vi "ChirpData.vi"(6 "element":T1, 8 "error in (no error)":errorcluster, 9 "NumDataPoints":u32, 10 "Work Unit Data Points":csg[](array[numeric]), 11 "SETI_LV_FPGA in":refnum<class "SETI_LV_FPGA.lvclass">) -> (0 "error out":errorcluster, 1 "NumDataPoints":u32, 2 "ChirpedData out":csg[](array[numeric]), 3 "SETI_LV_FPGA out":refnum<class "SETI_LV_FPGA.lvclass">)   [LabVIEW 2015, in "SETI_LV_FPGA.lvclass"]
uses:
  SETI_LV_FPGA.lvclass
  SETI_LV/TypeDefs/ChirpFFT Pairs.ctl
  SETI_LV/SETI_LV.lvlib
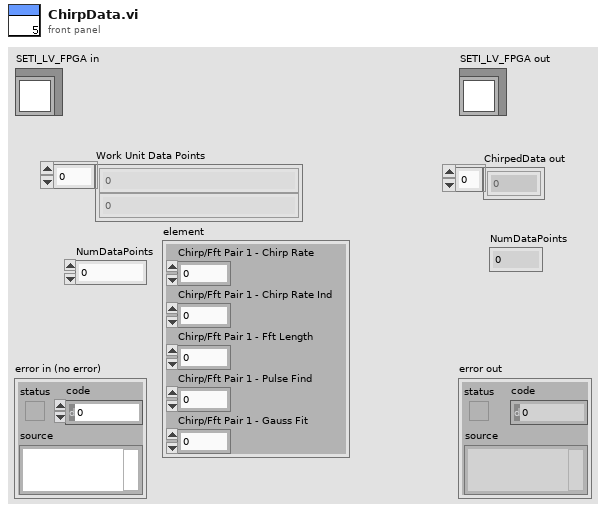
[diagram p1: front panel]
types:
  T1 = typedef "SETI_LV.lvlib/ChirpFFT Pairs.ctl" = cluster{"Chirp/Fft Pair 1 - Chirp Rate":dbl, "Chirp/Fft Pair 1 - Chirp Rate Ind":i32, "Chirp/Fft Pair 1 - Fft Length":i32, "Chirp/Fft Pair 1 - Pulse Find":i32, "Chirp/Fft Pair 1 - Gauss Fit":i32}
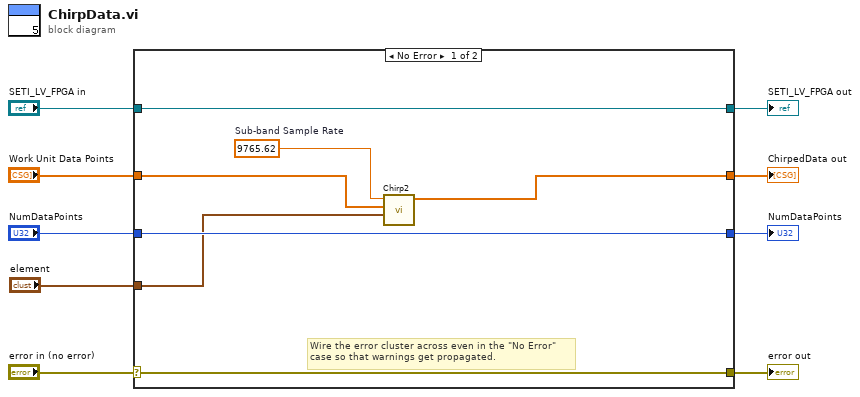
[diagram p0: block diagram]
diagram:
  n1 = case shown="No Error" "error in (no error)" {
    selector: "error in (no error)" -> [w16 w20]
    tunnel: [w16 w20] -> w8
    tunnel: [w12 w19] -> w6
    tunnel: "SETI_LV_FPGA in" -> [w12 w19]
    tunnel: [w10 w18] -> w3
    tunnel: "Work Unit Data Points" -> [w14 w18]
    tunnel: [w15 w17] -> w2
    tunnel: "NumDataPoints" -> [w15 w17]
    tunnel: "element" -> [w11 _]
    frame No Error {
      w13 = 9765.62  # Sub-band Sample Rate
      # "Wire the error cluster across even in the \"No Error\"\ncase so that warnings get propagated."
      n2 = call "Chirp2.vi"("Chirp Parameters (in)"=w11, "DataPoints (in)"=w14, "Sub-band Sample Rate (in)"=w13) -> ("ChirpedData (out)"=w10:csg[])  [unwired: 8 in]
    }
    frame Error {
    }
  }
  "error out" <- w8
  "SETI_LV_FPGA out" <- w6
  "ChirpedData out" <- w3
  "NumDataPoints" <- w2
